vi "valves_loadrings.vi"(0 "COM4 in":refnum<k24>, 1 "Frequency":dbl=1.0, 2 "Input solution":dbl=1.0, 3 "Cycles":i32=1, 4 "Rings to open":u32, 5 "error in":errorcluster) -> (6 "COM4 out":refnum<k24>, 8 "error out":errorcluster)   [LabVIEW 2018]
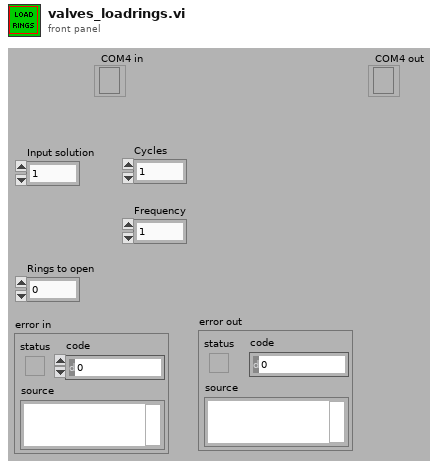
[diagram p1: front panel]
types:
  T1 = cluster{"Op A":u8[], "Op B":u8[], "Op C":u8[], "open":u8[], "L 3 A":u8[], "L 4 A 16":u8[], "F1 A":u8[], "L 4 A 34":u8[], "L 4 A 5":u8[], "FPw1 A":u8[], "L 2 A":u8[], "L 1 C FS":u8[], "L 2 C FS":u8[], "L 4 C 456 FS":u8[], "L 4 C 123 FS":u8[], "L 1 A":u8[], "L 1 C":u8[], "L 2 C":u8[], "L 4 C 456":u8[], "L 4 C 123":u8[], "FPw1 C":u8[], "F1 B":u8[], "F1 C":u8[], "F2 C":u8[], "F5 C":u8[]}
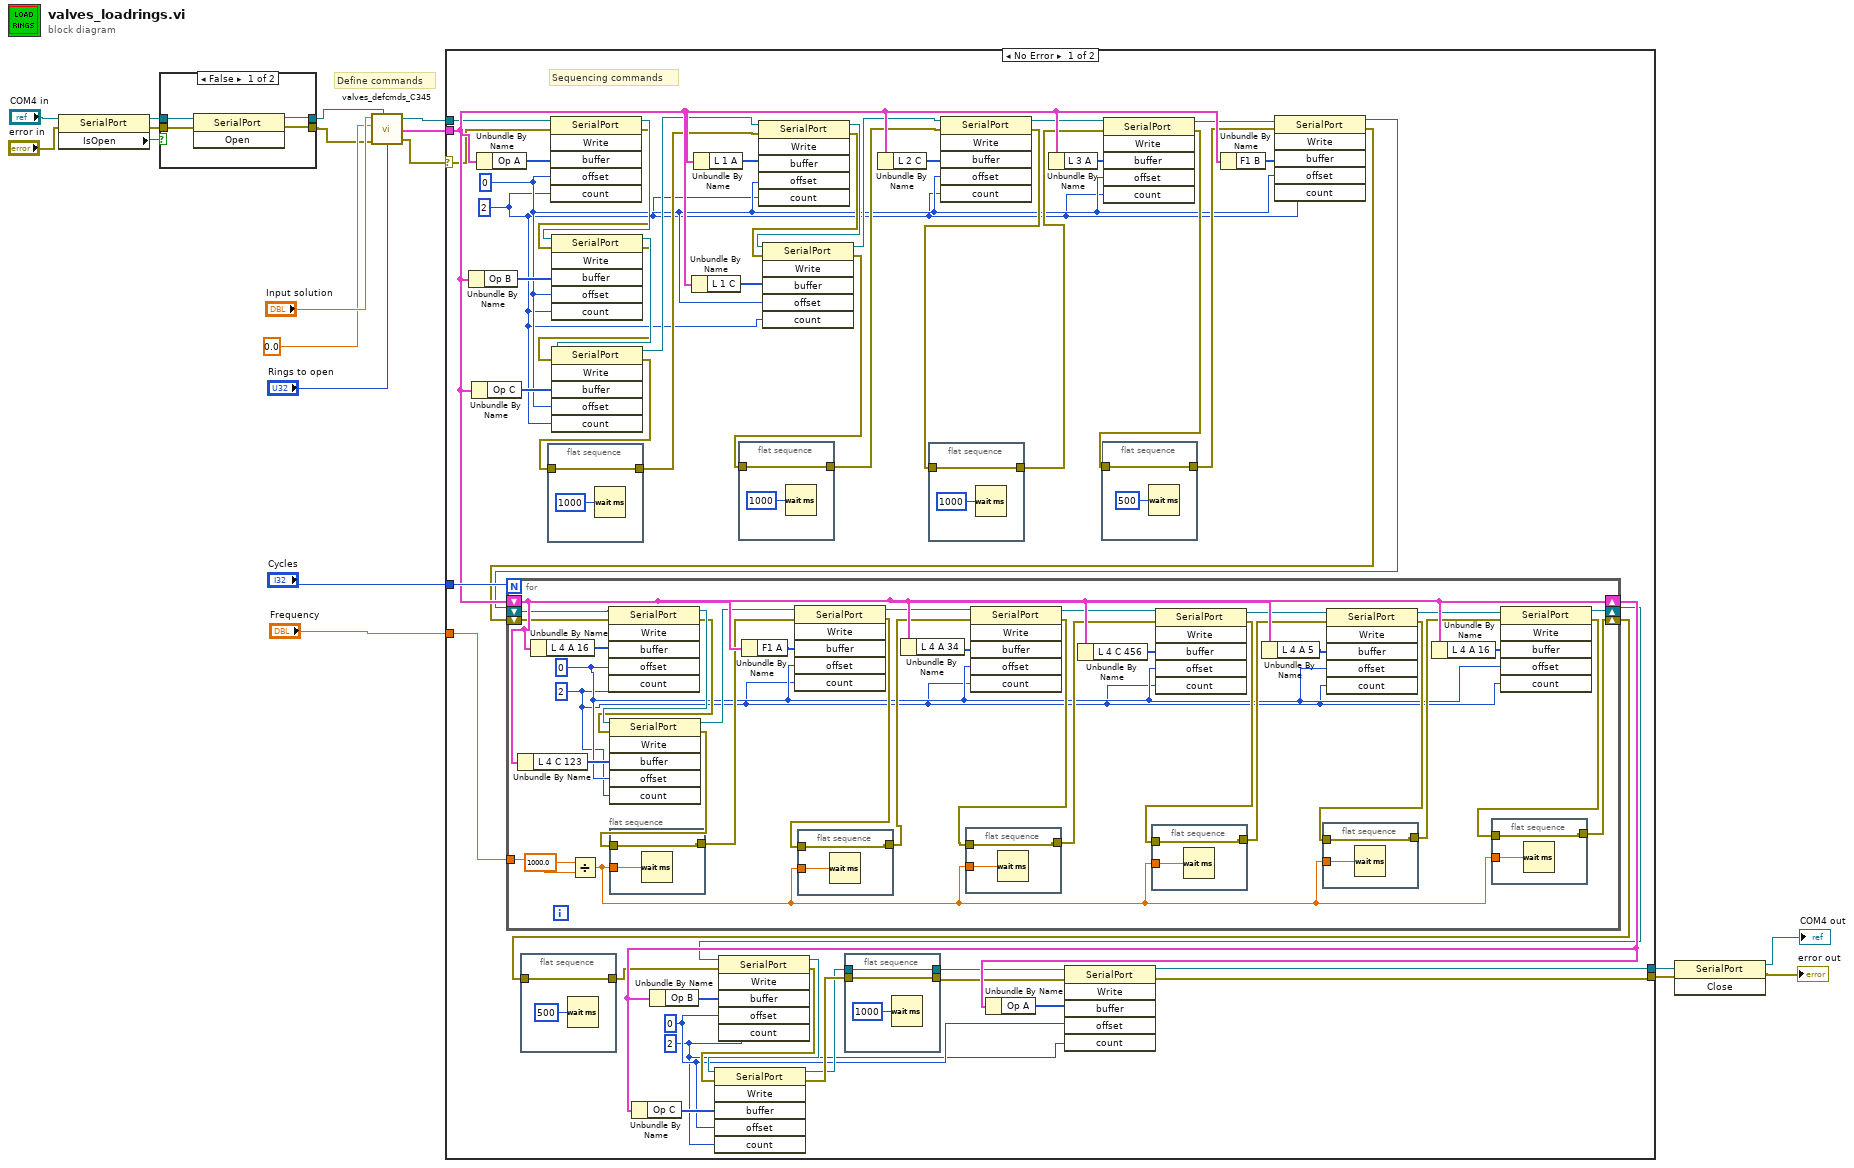
[diagram p0: block diagram]
diagram:
  # "Define commands"
  n1 = property class="SerialPort"(reference="COM4 in", error in="error in") -> (reference out=w9:refnum<k24>, error out=w10:errorcluster, "IsOpen"=w11:bool)
  n2 = case shown="False" w11 {
    tunnel: [w20 w25] -> w5
    tunnel: [w21 w24] -> w7
    tunnel: w10 -> [w22 w24]
    tunnel: w9 -> [w23 w25]
    frame False {
      n3 = invoke class="SerialPort" method="Open"(reference=w23, error in=w22) -> (reference out=w20:refnum<k24>, error out=w21:errorcluster)  [unwired: 1 in, 1 out]
    }
    frame True {
    }
  }
  n4 = call "valves_defcmds_C345.vi"("Input solution"="Input solution", "Add to C"=0.0, "Rings to open"="Rings to open", "error in"=w7, "COM4 in"=w5) -> ("COM4 out"=w16:refnum<k24>, "Commands out"=w18:T1, "error out"=w19:errorcluster)
  n5 = case shown="No Error" w19 {
    selector: w19 -> [w64 w139]
    tunnel: "Frequency" -> [w77 _]
    tunnel: "Cycles" -> [w76 _]
    tunnel: w16 -> [w72 w138]
    tunnel: [w31 w139] -> w4
    tunnel: [w30 w138] -> w3
    tunnel: w18 -> [w74 _]
    frame No Error {
      w26 = 2 ("count")
      w27 = 0 ("offset")
      w28 = 2 ("count")
      w29 = 0 ("offset")
      # "Sequencing commands"
      n6 = Unbundle By Name(w74) -> ("Op B"=w51:u8[])
      n7 = Unbundle By Name(w74) -> ("Op C"=w50:u8[])
      n8 = Unbundle By Name(w74) -> ("Op A"=w52:u8[])
      n9 = flat-sequence {
        tunnel: [w78] -> w41
        tunnel: w75 -> [w78]
        frame #0 {
          n10 = Wait (ms)(milliseconds to wait=u32 500) -> ()  [unwired: 1 out]
        }
      }
      n11 = flat-sequence {
        tunnel: [w136] -> w60
        tunnel: w61 -> [w136]
        frame #0 {
          n12 = Wait (ms)(milliseconds to wait=u32 1000) -> ()  [unwired: 1 out]
        }
      }
      n13 = invoke class="SerialPort" method="Write"(reference=w72, error in=w64, "buffer"=w52, "offset"=w29, "count"=w28) -> (reference out=w71:refnum<k24>, error out=w63:errorcluster)  [unwired: 1 in, 4 out]
      n14 = invoke class="SerialPort" method="Write"(reference=w71, error in=w63, "buffer"=w51, "offset"=w29, "count"=w28) -> (reference out=w70:refnum<k24>, error out=w62:errorcluster)  [unwired: 1 in, 4 out]
      n15 = invoke class="SerialPort" method="Write"(reference=w70, error in=w62, "buffer"=w50, "offset"=w29, "count"=w28) -> (reference out=w69:refnum<k24>, error out=w61:errorcluster)  [unwired: 1 in, 4 out]
      n16 = Unbundle By Name(w74) -> ("L 1 C"=w48:u8[])
      n17 = Unbundle By Name(w74) -> ("L 1 A"=w49:u8[])
      n18 = flat-sequence {
        tunnel: [w134] -> w57
        tunnel: w58 -> [w134]
        frame #0 {
          n19 = Wait (ms)(milliseconds to wait=u32 1000) -> ()  [unwired: 1 out]
        }
      }
      n20 = invoke class="SerialPort" method="Write"(reference=w69, error in=w60, "buffer"=w49, "offset"=w29, "count"=w28) -> (reference out=w68:refnum<k24>, error out=w59:errorcluster)  [unwired: 1 in, 4 out]
      n21 = invoke class="SerialPort" method="Write"(reference=w68, error in=w59, "buffer"=w48, "offset"=w29, "count"=w28) -> (reference out=w67:refnum<k24>, error out=w58:errorcluster)  [unwired: 1 in, 4 out]
      n22 = flat-sequence {
        tunnel: [w81] -> w32
        tunnel: w39 -> [w81]
        tunnel: w37 -> [w80]
        tunnel: [w80] -> w36
        frame #0 {
          n23 = Wait (ms)(milliseconds to wait=u32 1000) -> ()  [unwired: 1 out]
        }
      }
      n24 = Unbundle By Name(w74) -> ("L 2 C"=w47:u8[])
      n25 = flat-sequence {
        tunnel: [w132] -> w55
        tunnel: w56 -> [w132]
        frame #0 {
          n26 = Wait (ms)(milliseconds to wait=u32 1000) -> ()  [unwired: 1 out]
        }
      }
      n27 = invoke class="SerialPort" method="Write"(reference=w67, error in=w57, "buffer"=w47, "offset"=w29, "count"=w28) -> (reference out=w66:refnum<k24>, error out=w56:errorcluster)  [unwired: 1 in, 4 out]
      n28 = Unbundle By Name(w74) -> ("L 3 A"=w46:u8[])
      n29 = flat-sequence {
        tunnel: [w130] -> w53
        tunnel: w54 -> [w130]
        frame #0 {
          n30 = Wait (ms)(milliseconds to wait=u32 500) -> ()  [unwired: 1 out]
        }
      }
      n31 = invoke class="SerialPort" method="Write"(reference=w66, error in=w55, "buffer"=w46, "offset"=w29, "count"=w28) -> (reference out=w65:refnum<k24>, error out=w54:errorcluster)  [unwired: 1 in, 4 out]
      n32 = Unbundle By Name(w74) -> ("F1 B"=w45:u8[])
      n33 = invoke class="SerialPort" method="Write"(reference=w65, error in=w53, "buffer"=w45, "offset"=w29, "count"=w28) -> (reference out=w43:refnum<k24>, error out=w44:errorcluster)  [unwired: 1 in, 4 out]
      n34 = for {
        N: w76 -> [_]
        tunnel: w77 -> [w116]
        shift-right: [w92] -> w75
        shift-left: w44 -> [w105]
        shift-right: [w106] -> w42
        shift-left: w43 -> [w113]
        shift-right: [w114] -> w73
        shift-left: w74 -> [w114]
        w83 = 2 ("count")
        w84 = 0 ("offset")
        n35 = Unbundle By Name(w114) -> ("L 4 C 123"=w90:u8[])
        n36 = Unbundle By Name(w114) -> ("L 4 A 16"=w91:u8[])
        n37 = Divide(x=1000.0, y=w116) -> (x/y=w115:dbl)
        n38 = invoke class="SerialPort" method="Write"(reference=w113, error in=w105, "buffer"=w91, "offset"=w84, "count"=w83) -> (reference out=w112:refnum<k24>, error out=w104:errorcluster)  [unwired: 1 in, 4 out]
        n39 = invoke class="SerialPort" method="Write"(reference=w112, error in=w104, "buffer"=w90, "offset"=w84, "count"=w83) -> (reference out=w111:refnum<k24>, error out=w103:errorcluster)  [unwired: 1 in, 4 out]
        n40 = flat-sequence {
          tunnel: w115 -> [w123]
          tunnel: [w122] -> w102
          tunnel: w103 -> [w122]
          frame #0 {
            n41 = Wait (ms)(milliseconds to wait=w123) -> ()  [unwired: 1 out]
          }
        }
        n42 = Unbundle By Name(w114) -> ("F1 A"=w89:u8[])
        n43 = invoke class="SerialPort" method="Write"(reference=w111, error in=w102, "buffer"=w89, "offset"=w84, "count"=w83) -> (reference out=w110:refnum<k24>, error out=w101:errorcluster)  [unwired: 1 in, 4 out]
        n44 = flat-sequence {
          tunnel: w115 -> [w121]
          tunnel: w101 -> [w120]
          tunnel: [w120] -> w100
          frame #0 {
            n45 = Wait (ms)(milliseconds to wait=w121) -> ()  [unwired: 1 out]
          }
        }
        n46 = Unbundle By Name(w114) -> ("L 4 A 34"=w88:u8[])
        n47 = flat-sequence {
          tunnel: w115 -> [w125]
          tunnel: [w124] -> w98
          tunnel: w99 -> [w124]
          frame #0 {
            n48 = Wait (ms)(milliseconds to wait=w125) -> ()  [unwired: 1 out]
          }
        }
        n49 = invoke class="SerialPort" method="Write"(reference=w110, error in=w100, "buffer"=w88, "offset"=w84, "count"=w83) -> (reference out=w109:refnum<k24>, error out=w99:errorcluster)  [unwired: 1 in, 4 out]
        n50 = Unbundle By Name(w114) -> ("L 4 C 456"=w87:u8[])
        n51 = flat-sequence {
          tunnel: w115 -> [w127]
          tunnel: [w126] -> w96
          tunnel: w97 -> [w126]
          frame #0 {
            n52 = Wait (ms)(milliseconds to wait=w127) -> ()  [unwired: 1 out]
          }
        }
        n53 = invoke class="SerialPort" method="Write"(reference=w109, error in=w98, "buffer"=w87, "offset"=w84, "count"=w83) -> (reference out=w108:refnum<k24>, error out=w97:errorcluster)  [unwired: 1 in, 4 out]
        n54 = Unbundle By Name(w114) -> ("L 4 A 5"=w86:u8[])
        n55 = flat-sequence {
          tunnel: w115 -> [w129]
          tunnel: [w128] -> w94
          tunnel: w95 -> [w128]
          frame #0 {
            n56 = Wait (ms)(milliseconds to wait=w129) -> ()  [unwired: 1 out]
          }
        }
        n57 = invoke class="SerialPort" method="Write"(reference=w108, error in=w96, "buffer"=w86, "offset"=w84, "count"=w83) -> (reference out=w107:refnum<k24>, error out=w95:errorcluster)  [unwired: 1 in, 4 out]
        n58 = Unbundle By Name(w114) -> ("L 4 A 16"=w85:u8[])
        n59 = flat-sequence {
          tunnel: w115 -> [w119]
          tunnel: [w118] -> w92
          tunnel: w93 -> [w118]
          frame #0 {
            n60 = Wait (ms)(milliseconds to wait=w119) -> ()  [unwired: 1 out]
          }
        }
        n61 = invoke class="SerialPort" method="Write"(reference=w107, error in=w94, "buffer"=w85, "offset"=w84, "count"=w83) -> (reference out=w106:refnum<k24>, error out=w93:errorcluster)  [unwired: 1 in, 4 out]
      }
      n62 = Unbundle By Name(w73) -> ("Op C"=w35:u8[])
      n63 = Unbundle By Name(w73) -> ("Op B"=w34:u8[])
      n64 = invoke class="SerialPort" method="Write"(reference=w42, error in=w41, "buffer"=w34, "offset"=w27, "count"=w26) -> (reference out=w38:refnum<k24>, error out=w40:errorcluster)  [unwired: 1 in, 4 out]
      n65 = invoke class="SerialPort" method="Write"(reference=w38, error in=w40, "buffer"=w35, "offset"=w27, "count"=w26) -> (reference out=w37:refnum<k24>, error out=w39:errorcluster)  [unwired: 1 in, 4 out]
      n66 = Unbundle By Name(w73) -> ("Op A"=w33:u8[])
      n67 = invoke class="SerialPort" method="Write"(reference=w36, error in=w32, "buffer"=w33, "offset"=w27, "count"=w26) -> (reference out=w30:refnum<k24>, error out=w31:errorcluster)  [unwired: 1 in, 4 out]
    }
    frame Error {
    }
  }
  n68 = invoke class="SerialPort" method="Close"(reference=w3, error in=w4) -> (reference out=→"COM4 out":refnum<k24>, error out=→"error out":errorcluster)  [unwired: 1 in, 1 out]
